vi "USB send, no return.vi"(4 "Error in":errorcluster, 6 "Tx msg cluster":T1={"addr"=1, "cmd"="A", "data (float)"=0.0}, 7 "Port":refnum<visa-resource-name>) -> (0 "Error out":errorcluster, 3 "Port out":refnum<visa-resource-name>)   [LabVIEW 2017]
uses:
  ctls/USB Tx msg cluster.ctl
panel:
  out "Bytes sent":u32
  out "Write buffer":string
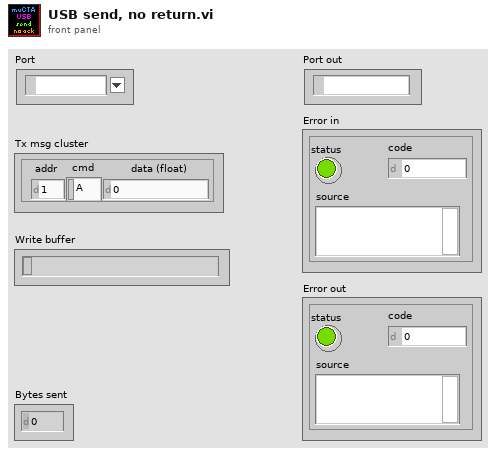
[diagram p1: front panel]
types:
  T1 = typedef "USB Tx msg cluster.ctl" = cluster{"addr":u8, "cmd":string, "data (float)":sgl}
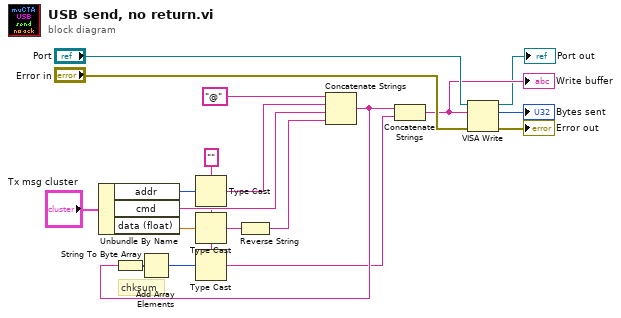
[diagram p0: block diagram]
diagram:
  w7 = ""
  # "chksum"
  n1 = Unbundle By Name("Tx msg cluster") -> ("addr"=w17:u8, "cmd"=w12:string, "data (float)"=w16:sgl)
  n2 = Type Cast(type=w7, x=w17) -> (*(type *) &x=w13:string)
  n3 = Type Cast(type=w7, x=w16) -> (*(type *) &x=w11:string)
  n4 = Reverse String(1:w11) -> (0:w1:string)
  n5 = Concatenate Strings("@", w13, w12, w1) -> (w9:string)
  n6 = String To Byte Array(string=w9) -> (unsigned byte array=w8:u8[])
  n7 = Add Array Elements(numeric array=w8) -> (sum=w6:u8)
  n8 = Type Cast(type=w7, x=w6) -> (*(type *) &x=w5:string)
  n9 = Concatenate Strings(w9, w5) -> (w10:string)
  "Write buffer" <- w10
  n10 = VISA Write(VISA resource name="Port", write buffer=w10, error in (no error)="Error in") -> (VISA resource name out=→"Port out":refnum<visa-resource-name>, return count=→"Bytes sent":u32, error out=→"Error out":errorcluster)
